vi "Draw Body Index Frame.vi"(8 "error in (no error)":errorcluster, 10 "Byte Array":u8[](array[numeric]), 11 "Image":T1) -> (0 "error out":errorcluster, 3 "Image Out":T1)   [LabVIEW 2014]
uses:
  <vilib>/vision/Image Controls.llb/IMAQ Image.ctl
  Frame Description FGV [Body Index].vi
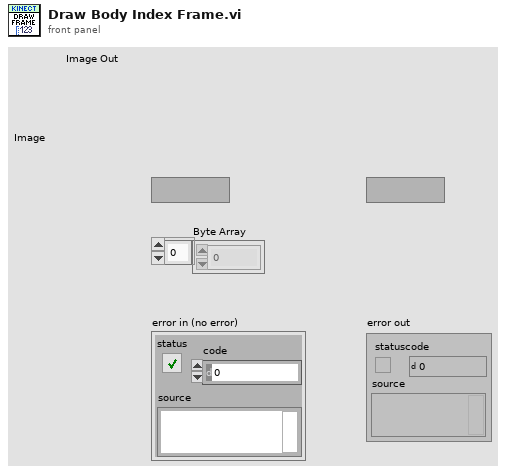
[diagram p1: front panel]
types:
  T1 = typedef "IMAQ Image.ctl" = refnum<image>
  T2 = typedef "FrameDescription.ctl" = cluster{"BytesPerPixel":u32, "DiagonalFieldOfView":sgl, "Height":i32, "HorizontalFieldOfView":sgl, "LengthInPixels":u32, "VerticalFieldOfView":sgl, "Width":i32}
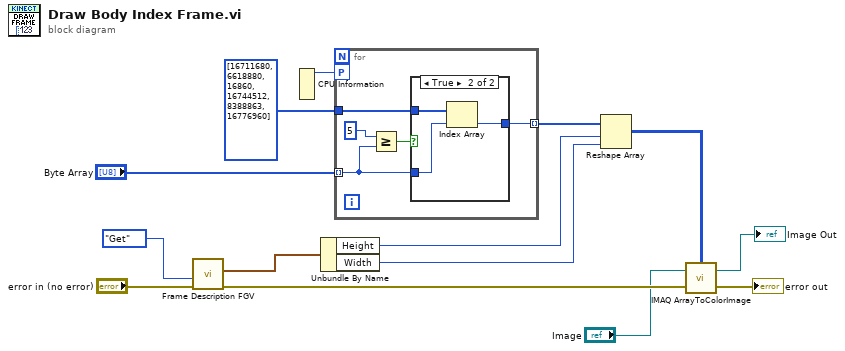
[diagram p0: block diagram]
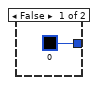
[diagram p2: hidden frame]
diagram:
  n1 = call-poly "Frame Description FGV.vi"("error in (no error)"="error in (no error)", "Command"=enum16{"Get", "Set"}."Get") -> ("error out"=w6:errorcluster, "FrameDescription"=w8:T2)  [unwired: 8 in]
  n2 = CPU Information() -> (4:w12:i32)  [unwired: 3 out]
  n3 = Unbundle By Name(w8) -> ("Height"=w11:i32, "Width"=w10:i32)
  n4 = for {
    tunnel: "Byte Array" -> [w16] mode=indexing
    tunnel: u32[] [16711680, 6618880, 16860, 16744512, 8388863, 16776960] -> [w19]
    tunnel: [w15] -> w9 mode=indexing
    workers-P: w12 -> [_]
    n5 = Greater Or Equal?(x=u8 5, y=w16) -> (x >= y?=w17:bool)
    n6 = case shown="True" w17 {
      tunnel: w19 -> [_ w23]
      tunnel: w16 -> [_ w22]
      tunnel: [u32 0 w21] -> w15
      frame False {
      }
      frame True {
        n7 = Index Array(array=w23, index=w22) -> (element=w21:u32)
      }
    }
  }
  n8 = Reshape Array(w9, w11, w10) -> (w7:u32[][])
  n9 = call "IMAQ ArrayToColorImage"("Image Pixels (U32)"=w7, "Image"="Image", "error in (no error)"=w6) -> ("Image Out"=→"Image Out":T1, "error out"=→"error out":errorcluster)  [unwired: 2 in]
